vi "GFITS_ParsePostProc.vi"(10 "postproc in":string) -> (2 "postproc out":string)   [LabVIEW 2016]
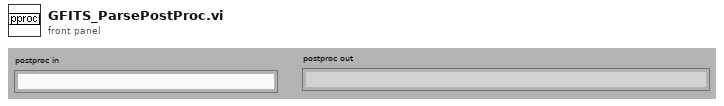
[diagram p1: front panel]
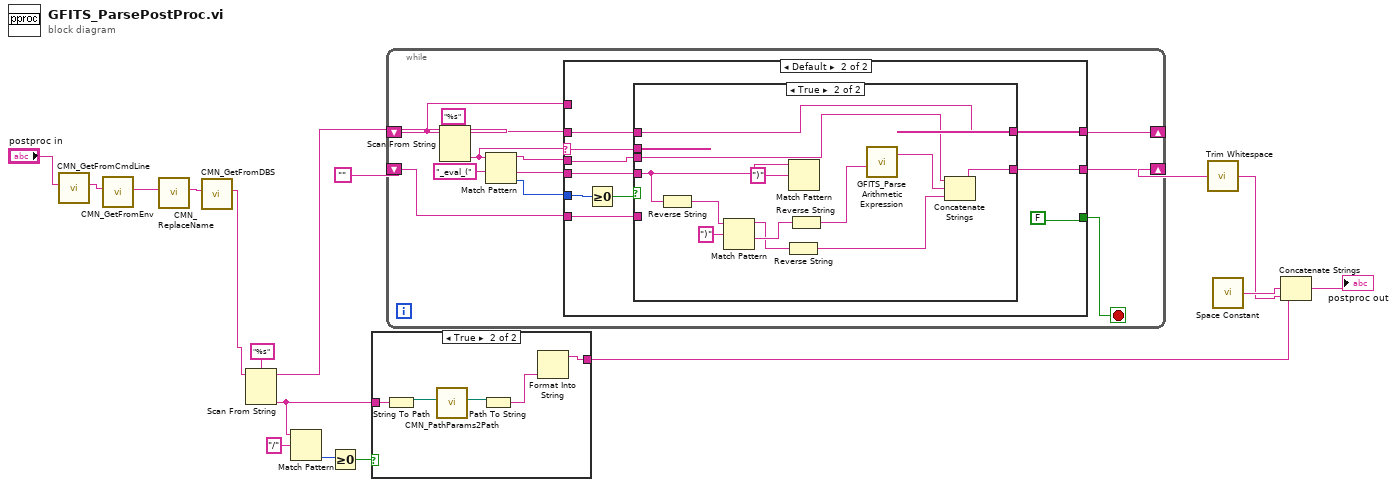
[diagram p0: block diagram]
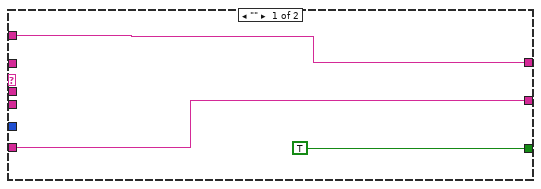
[diagram p3: hidden frame]
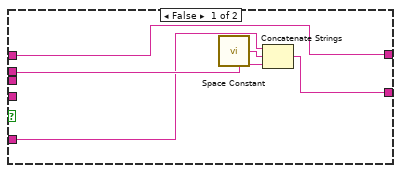
[diagram p4: hidden frame]
diagram:
  n1 = call "CMN_GetFromCmdLine.vi"("str in"="postproc in") -> ("str out"=w9:string)  [unwired: 10 out]
  n2 = call "CMN_GetFromEnv.vi"("str in"=w9) -> ("str out"=w7:string)  [unwired: 10 out]
  n3 = call "CMN_ReplaceName.vi"("name in"=w7) -> ("name out"=w15:string)  [unwired: 1 in, 9 out]
  n4 = call "CMN_GetFromDBS.vi"("str in"=w15) -> ("str out"=w6:string)  [unwired: 10 out]
  n5 = Scan From String(format string="%s", input string=w6) -> (remaining string=w1:string, output 1=w5:string)  [unwired: 2 in, 3 out]
  n6 = Match Pattern(string=w5, regular expression="/") -> (offset past match=w3:i32)  [unwired: 4 out]
  n7 = Greater Or Equal To 0?(x=w3) -> (x >= 0?=w2:bool)
  n8 = case shown="True" w2 {
    tunnel: [w18 w20] -> w16
    tunnel: w5 -> [w18 w19]
    frame False {
    }
    frame True {
      n9 = String To Path(string=w19) -> (path=w23:path)
      n10 = call "CMN_PathParams2Path.vi"("Path In"=w23) -> ("Path out"=w22:path)  [unwired: 2 in, 8 out]
      n11 = Path To String(path=w22) -> (string=w21:string)
      n12 = Format Into String(w21) -> (resulting string=w20:string)  [unwired: 3 in, 1 out]
    }
  }
  n13 = while {
    shift-right: [w32] -> _
    shift-left: w1 -> [w25]
    shift-right: [w27] -> w12
    shift-left: "" -> [w28]
    stop <- w30 stop-if-true
    n14 = Scan From String(format string="%s", input string=w25) -> (remaining string=w26:string, output 1=w31:string)  [unwired: 2 in, 3 out]
    n15 = Match Pattern(string=w31, regular expression="_eval_(") -> (before substring=w24:string, after substring=w29:string, offset past match=w33:i32)  [unwired: 2 out]
    n16 = case shown="Default" w31 {
      selector: w31 -> [_ w43]
      tunnel: w33 -> [_ w48]
      tunnel: [w37 w46] -> w32
      tunnel: [TRUE FALSE] -> w30
      tunnel: w29 -> [_ w44]
      tunnel: w28 -> [w36 w42]
      tunnel: [w36 w41] -> w27
      tunnel: w26 -> [_ w40]
      tunnel: w25 -> [w37 _]
      tunnel: w24 -> [_ w39]
      frame "" {
      }
      frame Default {
        n17 = Greater Or Equal To 0?(x=w48) -> (x >= 0?=w47:bool)
        n18 = case shown="True" w47 {
          tunnel: w43 -> [w53 _]
          tunnel: [w49 w64] -> w46
          tunnel: w44 -> [_ w60]
          tunnel: w42 -> [w51 _]
          tunnel: [w50 w62] -> w41
          tunnel: w40 -> [w49 w64]
          tunnel: w39 -> [_ w63]
          frame False {
            n19 = call <vilib>:"Space Constant.vi"() -> ("String"=w52:string)
            n20 = Concatenate Strings(w51, w52, w53) -> (w50:string)
          }
          frame True {
            n21 = Reverse String(1:w60) -> (0:w59:string)
            n22 = Match Pattern(string=w59, regular expression=")") -> (before substring=w56:string, after substring=w57:string)  [unwired: 3 out]
            n23 = Reverse String(1:w56) -> (0:w55:string)
            n24 = Match Pattern(string=w60, regular expression=")") -> ()  [unwired: 5 out]
            n25 = Reverse String(1:w57) -> (0:w54:string)
            n26 = call "GFITS_Parse Arithmetic Expression.vi"("Arithmetic Expression"=w54) -> ("string_result"=w61:string)  [unwired: 4 out]
            n27 = Concatenate Strings(w63, w61, w55) -> (w62:string)
          }
        }
      }
    }
  }
  n28 = call <vilib>:"Trim Whitespace.vi"("string"=w12) -> ("trimmed string"=w10:string)  [unwired: 1 in]
  n29 = call <vilib>:"Space Constant.vi"() -> ("String"=w11:string)
  n30 = Concatenate Strings(w16, w11, w10) -> (→"postproc out":string)
